vi "sendCloseLog.vi"(8 "error in (no error)":errorcluster, 11 "Source":string) -> (0 "error out":errorcluster)   [LabVIEW 2017, in "loggingModule.lvlib"]
uses:
  loggingModule.lvlib
  Queue/TypeDefs/message.ctl
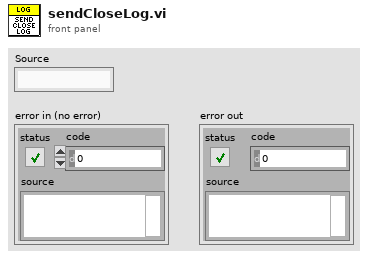
[diagram p1: front panel]
types:
  T1 = typedef "loggingModule.lvlib/message.ctl" = cluster{"calling module":string, "message":string, "data":variant}
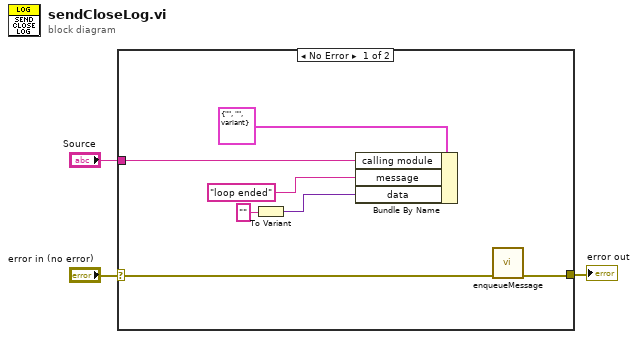
[diagram p0: block diagram]
diagram:
  n1 = case shown="No Error" "error in (no error)" {
    selector: "error in (no error)" -> [w5 w11]
    tunnel: [w6 w11] -> w3
    tunnel: "Source" -> [w4 _]
    frame No Error {
      n2 = To Variant(anything="") -> (Variant=w10:variant)
      n3 = Bundle By Name(cluster=T1 {"calling module"="", "message"="", "data"=variant} ("message in"), "calling module"=w4, "message"="loop ended", "data"=w10) -> ()  [unwired: 1 out]
      n4 = call "enqueueMessage.vi"("error in (no error)"=w5) -> ("error out"=w6:errorcluster)  [unwired: 10 in]
    }
    frame Error {
    }
  }
  "error out" <- w3
